vi "FTP_Read.vi"(4 "error In":errorcluster, 5 "expected class":T1(ring)=enum."500 - Permanent", 7 "connection ID":refnum<k5>) -> (0 "error out":errorcluster, 1 "Good Reply?":bool, 2 "reply string":string, 3 "connection ID out":refnum<k5>)   [LabVIEW 2012]
uses:
  <userlib>/BotSpeak/Devices/EvalRIO/FTPCodes/FTPGlobals.vi
panel:
  out "reply code":i32
  in  "Num Retries":i32=5
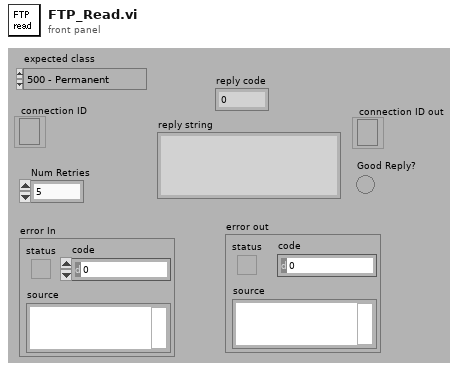
[diagram p1: front panel]
types:
  T1 = enum16{"unknown", "100 + Prelim", "200 + ", "300 + Intermed", "400 - Transient", "500 - Permanent"}
  T2 = enum16{"Standard", "Buffered", "CRLF", "Immediate"}
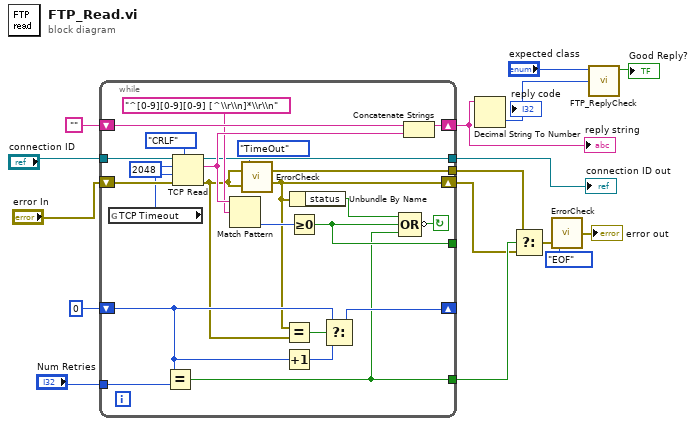
[diagram p0: block diagram]
diagram:
  n1 = while {
    tunnel: [w29] -> _
    tunnel: [w30] -> w4
    tunnel: "connection ID" -> [w35]
    shift-left: "error In" -> [w36]
    shift-right: [w19] -> w12
    shift-left: "" -> [w33]
    shift-right: [w32] -> w10
    shift-right: [w24] -> _
    shift-left: 0 -> [w23]
    tunnel: "Num Retries" -> [w22]
    tunnel: [w21] -> w13
    tunnel: [w20] -> w11
    stop <- w38 continue-if-true
    n2 = global read "FTPGlobals.vi" "TCP Timeout"() -> (w17:i32)
    n3 = Equal?(x=w23, y=w22) -> (x = y?=w21:bool)
    n4 = TCP Read(connection ID=w35, bytes to read=2048, error in (no error)=w36, 7:T2."CRLF" ("mode (standard)"), 9:w17) -> (connection ID out=w30:refnum<k5>, data out=w34:string, error out=w20:errorcluster)
    n5 = Match Pattern(string=w34, regular expression="^[0-9][0-9][0-9] [^\\r\\n]*\\r\\n") -> (offset past match=w37:i32)  [unwired: 4 out]
    n6 = call <userlib>:"ErrorCheck.vi"("error in (no error)"=w20, "Err Check"=enum16{"TimeOut", "EOF"}."TimeOut") -> ("error out"=w19:errorcluster)
    n7 = Equal?(x=w19, y=w20) -> (x = y?=w26:bool)
    n8 = Increment(x=w23) -> (x+1=w25:i32)
    n9 = Greater Or Equal To 0?(x=w37) -> (x >= 0?=w29:bool)
    n10 = Unbundle By Name(w19) -> ("status"=w39:bool)
    n11 = Select(t=w23, s=w26, f=w25) -> (s? t:f=w24:i32)
    n12 = Compound Arithmetic op=OR(w39, w29, w21) -> (invert w38:bool)
    n13 = Concatenate Strings(w33, w34) -> (w32:string)
  }
  "reply string" <- w10
  "connection ID out" <- w4
  n14 = Decimal String To Number(string=w10) -> (number=w3:i32)  [unwired: 3 out]
  "reply code" <- w3
  n15 = Select(t=w11, s=w13, f=w12) -> (s? t:f=w14:errorcluster)
  n16 = call <userlib>:"ErrorCheck.vi"("error in (no error)"=w14, "Err Check"=enum16{"TimeOut", "EOF"}."EOF") -> ("error out"=→"error out":errorcluster)
  n17 = call <userlib>:"FTP_ReplyCheck.vi"("expected class"="expected class", "reply"=w3) -> ("match"=→"Good Reply?":bool)  [unwired: 4 out]
